vi "SDCP - Write Parameter To Frame.vi"(3 "error in (no error)":errorcluster, 4 "Value":dbl, 5 "Parameter Name":string) -> (0 "error out":errorcluster, 2 "Encoded message frame":u8[](array[numeric]))   [LabVIEW 2020]
uses:
  Typedefs/SDCP - Standard Message Frame Parameters - FGV - commands.ctl
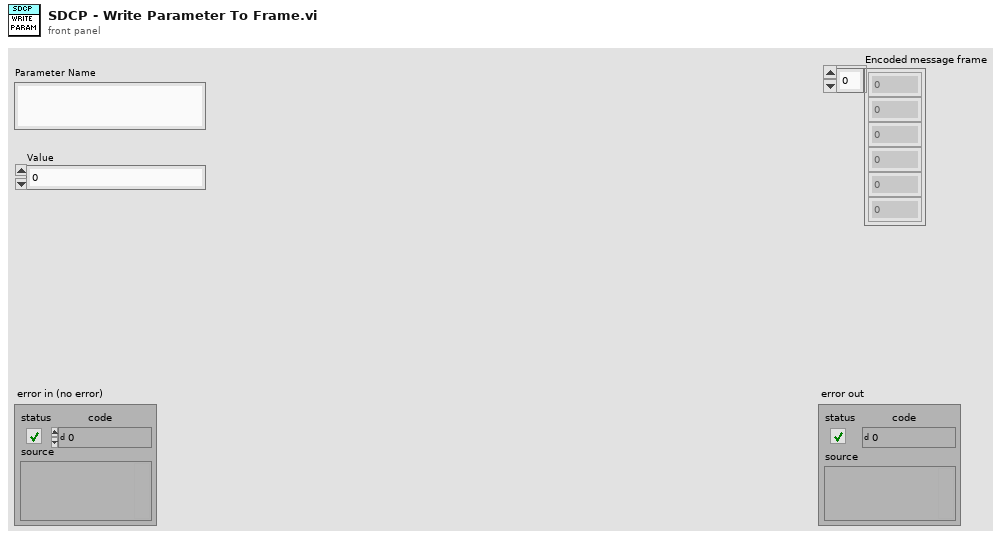
[diagram p1: front panel]
types:
  T1 = typedef "SDCP - Standard Message Frame Parameters - FGV - commands.ctl" = enum16{"Write descriptors", "Read descriptors", "Read values", "Load parameters from file", "Write values", "Read all descriptors"}
  T2 = typedef "SDCP - SMF parameter descriptors.ctl" = cluster{"Frame name":string, "Frame ID":i32, "Data type":string, "Start Position":i32, "Length":i32, "Factor":dbl, "Offset":dbl, "Parameter name":string, "Value":string}
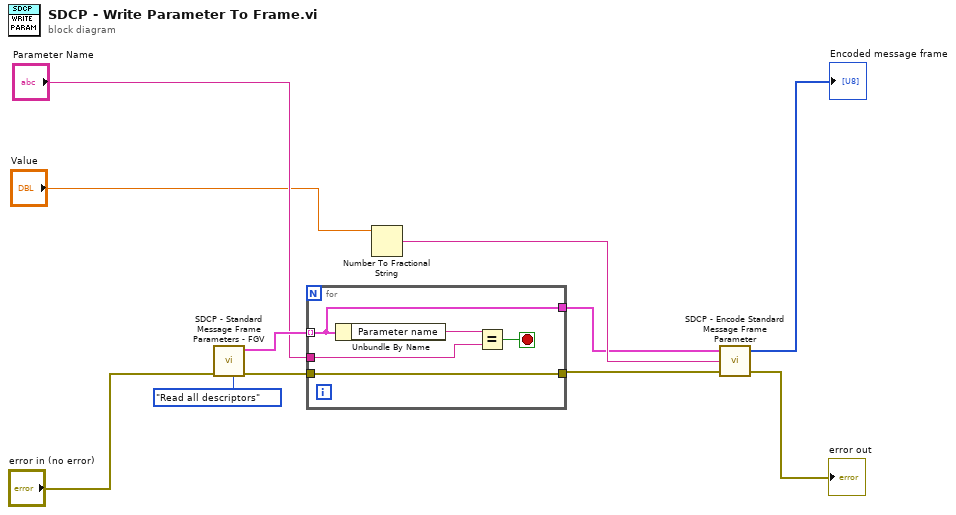
[diagram p0: block diagram]
diagram:
  n1 = call "SDCP - Standard Message Frame Parameters - FGV.vi"("error in (no error)"="error in (no error)", "Command"=SDCP_-_Standard_Message_Frame_Parameters_-_FGV_-_commands."Read all descriptors") -> ("SMF Parameters descriptors out"=w8:T2[], "error out"=w9:errorcluster)  [unwired: 5 in]
  n2 = for {
    tunnel: w9 -> [w16]
    tunnel: w8 -> [w12] mode=indexing
    tunnel: [w16] -> w6
    tunnel: "Parameter Name" -> [w14]
    tunnel: [w12] -> w3
    stop <- w13 stop-if-true
    n3 = Unbundle By Name(w12) -> ("Parameter name"=w15:string)
    n4 = Equal?(x=w15, y=w14) -> (x = y?=w13:bool)
  }
  n5 = Number To Fractional String(number="Value") -> (F-format string=w4:string)  [unwired: 3 in]
  n6 = call "SDCP - Encode Standard Message Frame Parameter.vi"("error in (no error)"=w6, "Value in"=w4, "SMF descriptor in"=w3) -> ("error out"=→"error out":errorcluster, "Encoded message frame"=→"Encoded message frame":u8[])  [unwired: 1 in]
